vi "ultrasonic PING.vi"(7 "DIO Refnum":refnum<k21>="ConnectorA/DIO7", 8 "DIR":bool, 9 "OUT":bool, 10 "timeout(us)":i32, 11 "F selection":bool) -> (1 "IN":bool, 3 "ultrasonic output":i32)   [LabVIEW 2019]
uses:
  <vilib>/rvi/eio/common/nirviEmuTemplateMethod_errors.vi
  <vilib>/eio/EIOMethodNode/EIOMethodNode.xnode
  <vilib>/eio/EIONode/EIONode.xnode
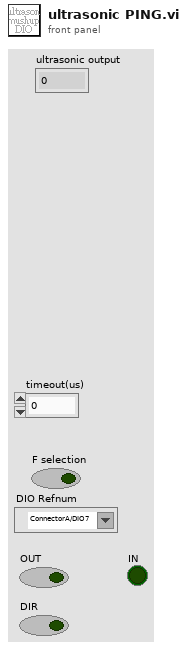
[diagram p1: front panel]
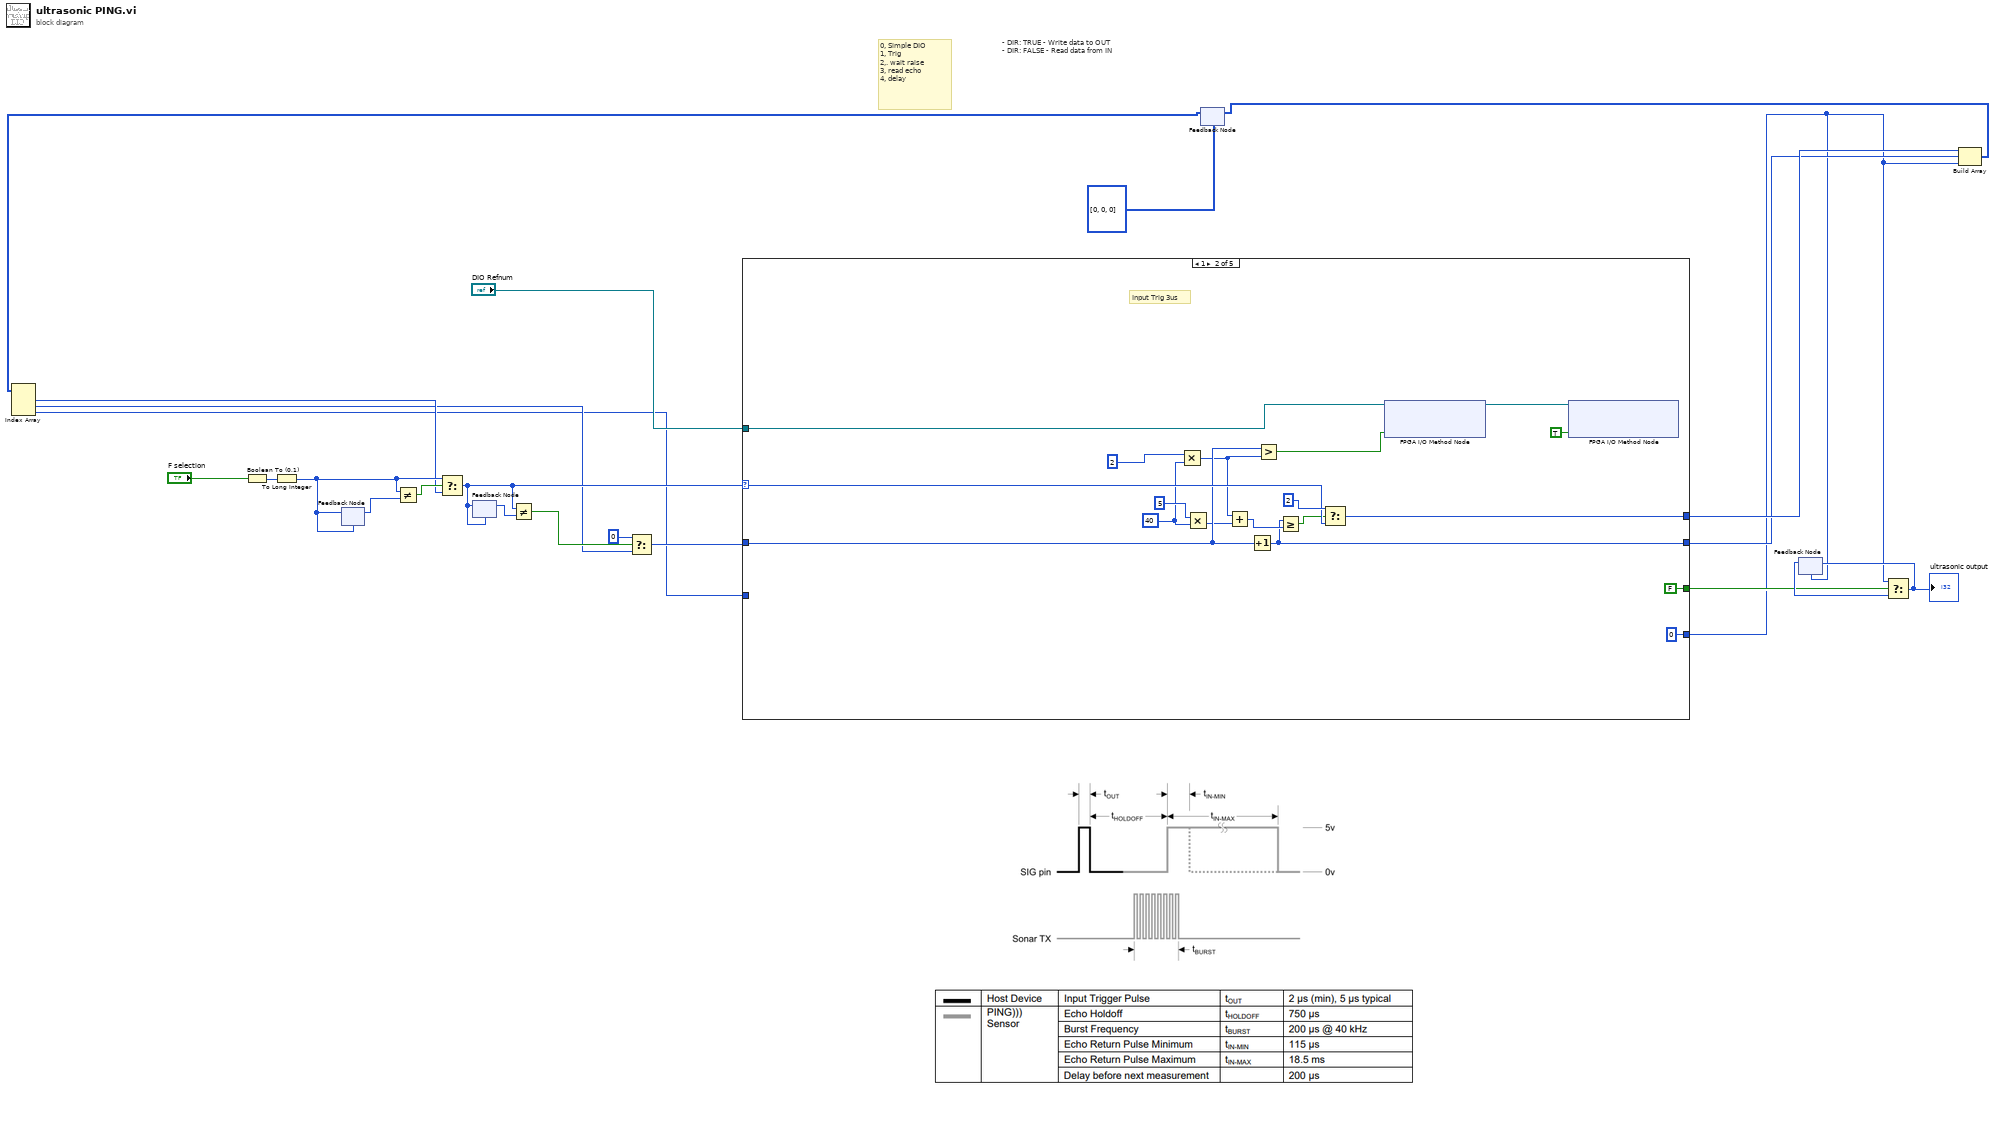
[diagram p0: block diagram]
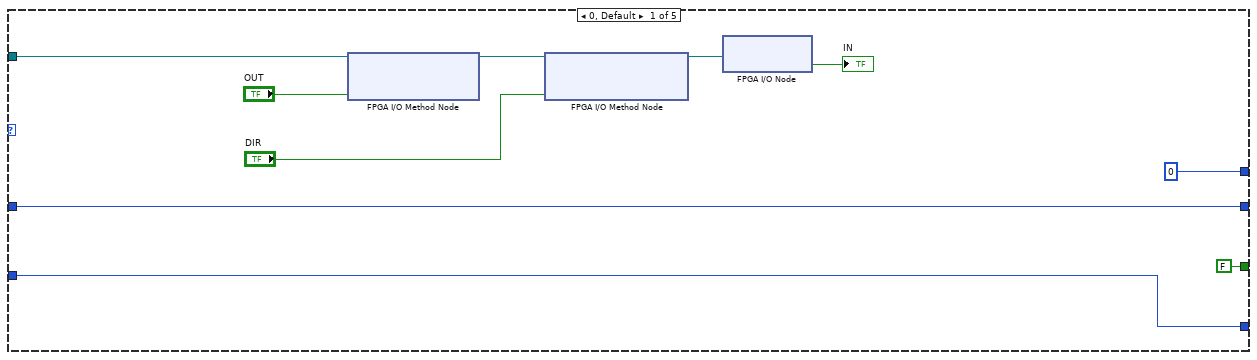
[diagram p2: hidden frame]
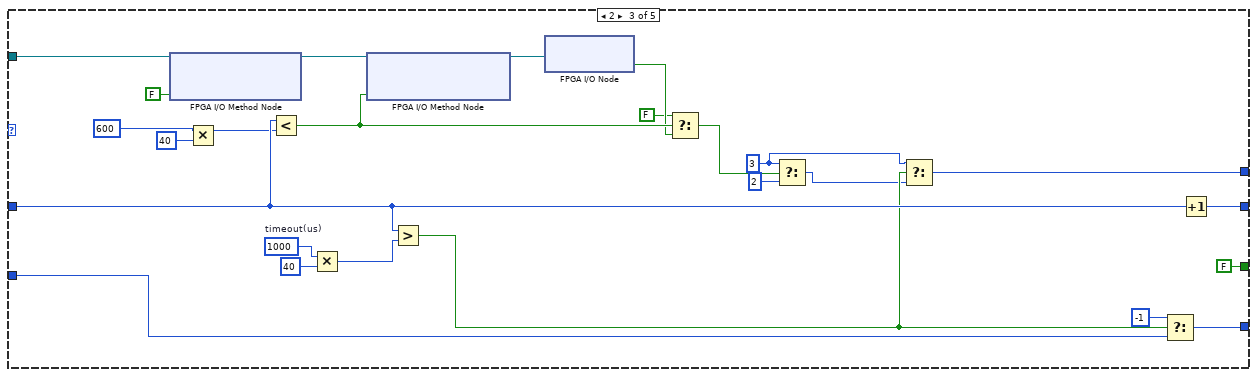
[diagram p3: hidden frame]
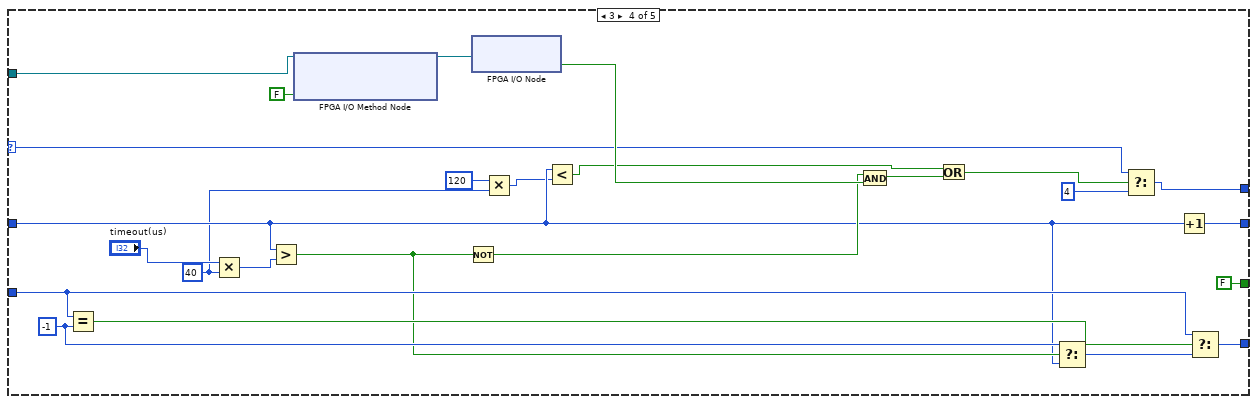
[diagram p4: hidden frame]
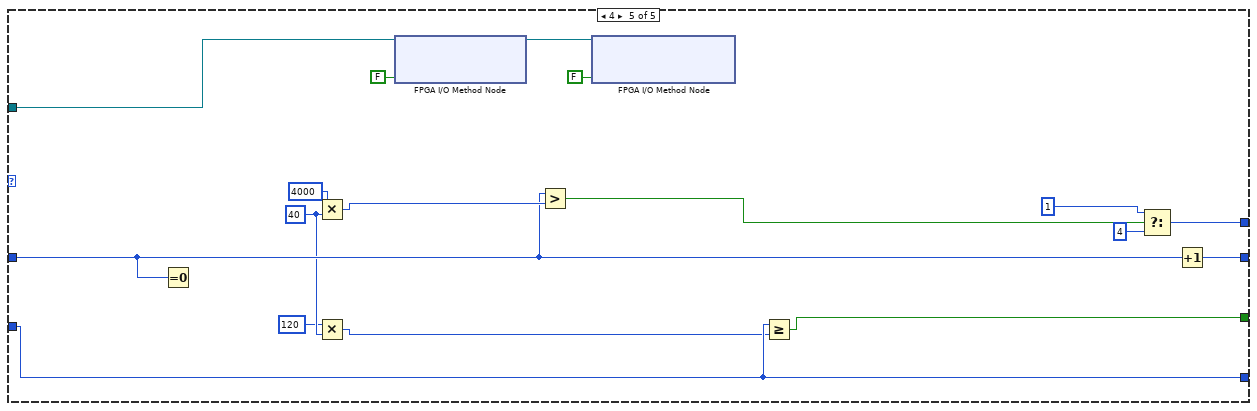
[diagram p5: hidden frame]
diagram:
  # "- DIR: TRUE - Write data to OUT\n- DIR: FALSE - Read data from IN"
  # "0, Simple DIO\n1, Trig\n2,. wait raise\n3, read echo\n4, delay"
  n1 = Boolean To (0,1)(Boolean="F selection") -> (0, 1=w14:i16)
  n2 = To Long Integer(number=w14) -> (32bit integer=w7:i32)
  n3 = feedback-in #1(w7) -> ()
  n4 = feedback #1(w7) -> (w23:i32)
  n5 = Not Equal?(x=w7, y=w23) -> (x != y?=w22:bool)
  n6 = feedback #2(i32[] [0, 0, 0]) -> (w2:i32[])
  n7 = Index Array(array=w2) -> (element #1=w6:i32, element #2=w5:i32, element #3=w4:i32)  [unwired: 3 in]
  n8 = Select(t=w7, s=w22, f=w6) -> (s? t:f=w19:i32)
  n9 = feedback-in #3(w19) -> ()
  n10 = feedback #3(w19) -> (w18:i32)
  n11 = Not Equal?(x=w19, y=w18) -> (x != y?=w17:bool)
  n12 = Select(t=0, s=w17, f=w5) -> (s? t:f=w20:i32)
  n13 = case shown="1" w19 {
    selector: w19 -> [_ w49 _ w94 _]
    tunnel: [0 w51 w55 w96 w115] -> w10
    tunnel: w20 -> [w25 w42 w61 w82 w108]
    tunnel: [w25 w35 w68 w98 w118] -> w9
    tunnel: "DIO Refnum" -> [w27 w47 w74 w100 w110]
    tunnel: w4 -> [w26 _ w63 w91 w106]
    tunnel: [w26 0 ("t") w62 w93 w106] -> w8
    tunnel: [FALSE FALSE FALSE FALSE w102] -> w11
    frame 0, Default {
      n14 = xnode "FPGA I/O Method Node"("FPGA I/O In"=w27, "Data"="OUT") -> ("FPGA I/O Out"=w30:refnum<k21>)
      n15 = xnode "FPGA I/O Method Node"("FPGA I/O In"=w30, "Enable"="DIR") -> ("FPGA I/O Out"=w29:refnum<k21>)
      n16 = xnode "FPGA I/O Node"("FPGA I/O In"=w29) -> ("I/O Item"=→"IN":bool)  [unwired: 1 out]
    }
    frame 1 {
      w38 = 40 ("y")
      # "Input Trig 3us"
      n17 = Multiply(x=2 ("y"), y=w38) -> (x*y=w34:i32)
      n18 = Multiply(x=5 ("y"), y=w38) -> (x*y=w37:i32)
      n19 = Add(x=w34, y=w37) -> (x+y=w36:i32)
      n20 = Increment(x=w42) -> (x+1=w35:i32)
      n21 = Greater?(x=w42, y=w34) -> (0:w41:bool)
      n22 = Greater Or Equal?(x=w35, y=w36) -> (x >= y?=w46:bool)
      n23 = Select(t=2, s=w46, f=w49) -> (s? t:f=w51:i32)
      n24 = xnode "FPGA I/O Method Node"("FPGA I/O In"=w47, "Data"=w41) -> ("FPGA I/O Out"=w48:refnum<k21>)
      n25 = xnode "FPGA I/O Method Node"("FPGA I/O In"=w48, "Enable"=TRUE) -> ()  [unwired: 1 out]
    }
    frame 2 {
      w65 = 1000  # timeout(us)
      w57 = 3
      n26 = xnode "FPGA I/O Method Node"("FPGA I/O In"=w74, "Data"=FALSE) -> ("FPGA I/O Out"=w76:refnum<k21>)
      n27 = Multiply(x=600 ("y"), y=40) -> (x*y=w54:i32)
      n28 = Less?(x=w61, y=w54) -> (x < y?=w71:bool)
      n29 = Multiply(x=w65, y=40) -> (x*y=w60:i32)
      n30 = xnode "FPGA I/O Method Node"("FPGA I/O In"=w76, "Enable"=w71) -> ("FPGA I/O Out"=w75:refnum<k21>)
      n31 = Greater?(x=w61, y=w60) -> (0:w58:bool)
      n32 = xnode "FPGA I/O Node"("FPGA I/O In"=w75) -> ("I/O Item"=w70:bool)  [unwired: 1 out]
      n33 = Select(t=FALSE, s=w71, f=w70) -> (s? t:f=w67:bool)
      n34 = Select(t=w57, s=w67, f=2) -> (s? t:f=w56:i32)
      n35 = Select(t=w57, s=w58, f=w56) -> (s? t:f=w55:i32)
      n36 = Select(t=-1, s=w58, f=w63) -> (s? t:f=w62:i32)
      n37 = Increment(x=w61) -> (x+1=w68:i32)
    }
    frame 3 {
      w80 = 40 ("y")
      w87 = -1 ("y")
      n38 = Equal?(x=w91, y=w87) -> (x = y?=w92:bool)
      n39 = Multiply(x="timeout(us)", y=w80) -> (x*y=w89:i32)
      n40 = Greater?(x=w82, y=w89) -> (0:w86:bool)
      n41 = xnode "FPGA I/O Method Node"("FPGA I/O In"=w100, "Enable"=FALSE) -> ("FPGA I/O Out"=w101:refnum<k21>)
      n42 = Not(x=w86) -> (.not. x?=w85:bool)
      n43 = xnode "FPGA I/O Node"("FPGA I/O In"=w101) -> ("I/O Item"=w95:bool)  [unwired: 1 out]
      n44 = Multiply(x=120, y=w80) -> (x*y=w81:i32)
      n45 = Less?(x=w82, y=w81) -> (x < y?=w78:bool)
      n46 = And(x=w85, y=w95) -> (x .and. y?=w84:bool)
      n47 = Or(x=w78, y=w84) -> (x .or. y?=w83:bool)
      n48 = Select(t=w87, s=w86, f=w82) -> (s? t:f=w88:i32)
      n49 = Select(t=w94, s=w83, f=4) -> (s? t:f=w96:i32)
      n50 = Increment(x=w82) -> (x+1=w98:i32)
      n51 = Select(t=w91, s=w92, f=w88) -> (s? t:f=w93:i32)
    }
    frame 4 {
      w105 = 40 ("y")
      n52 = Equal To 0?(x=w108) -> ()  [unwired: 1 out]
      n53 = Multiply(x=4000, y=w105) -> (x*y=w116:i32)
      n54 = Multiply(x=120, y=w105) -> (x*y=w103:i32)
      n55 = xnode "FPGA I/O Method Node"("FPGA I/O In"=w110, "Data"=FALSE) -> ("FPGA I/O Out"=w112:refnum<k21>)
      n56 = Greater?(x=w108, y=w116) -> (0:w114:bool)
      n57 = xnode "FPGA I/O Method Node"("FPGA I/O In"=w112, "Enable"=FALSE) -> ()  [unwired: 1 out]
      n58 = Greater Or Equal?(x=w106, y=w103) -> (x >= y?=w102:bool)
      n59 = Select(t=1, s=w114, f=4) -> (s? t:f=w115:i32)
      n60 = Increment(x=w108) -> (x+1=w118:i32)
    }
  }
  n61 = feedback #4(w8) -> (w13:i32)
  n62 = Select(t=w8, s=w11, f=w13) -> (s? t:f=w12:i32)
  "ultrasonic output" <- w12
  n63 = feedback-in #4(w12) -> ()
  n64 = Build Array(w10, w9, w8) -> (w3:i32[])
  n65 = feedback-in #2(w3) -> ()
